vi "ArmIncrementR-L-E.vi"(9 "AddE":dbl, 10 "AddL":dbl, 11 "AddR":dbl) -> ()   [LabVIEW 2020]
doc: "Increment Rotate, Lift, Extend values\n\nInput:\n--AddR--Double--how much to increment Rotate\n--AddL--Double--how much to increment Lift\n--AddE--Double--how much to increment Extend"
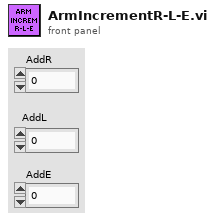
[diagram p1: front panel]
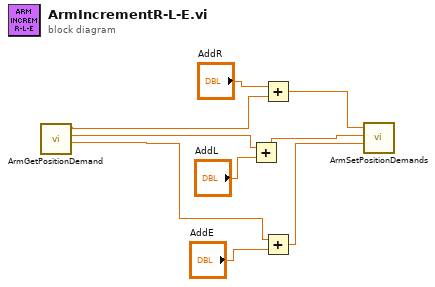
[diagram p0: block diagram]
diagram:
  n1 = call "ArmGetPositionDemand.vi"() -> ("ExtendPositonDemand(in)"=w1:dbl, "LiftPositionDemand(d)"=w2:dbl, "RotatePositonDemand(d)"=w3:dbl)  [unwired: 9 in]
  n2 = Add(x=w2, y="AddL") -> (x+y=w5:dbl)
  n3 = Add(x="AddR", y=w3) -> (x+y=w6:dbl)
  n4 = Add(x=w1, y="AddE") -> (x+y=w4:dbl)
  n5 = call "ArmSetPositionDemands.vi"("SetExtendPositonDemand(in)"=w4, "SetLIftPostionDemand(d)"=w5, "SetRotatePostionDemand(d)"=w6) -> ()  [unwired: 9 in]
